vi "DeleteEmptyFolders.vi"() -> ()   [LabVIEW 2020]
uses:
  <resource>/dialog/lvconfig.llb/LV Config Read String.vi
  <userlib>/_MGI/Application Control/MGI Gray if/MGI Gray if False.vi
panel:
  in  "ButtonDelete":bool
  out "FoldersToExclude":string[](array[string])
  out "ContainsEmptyFolder(s)?":bool
  in  "Root Path":path
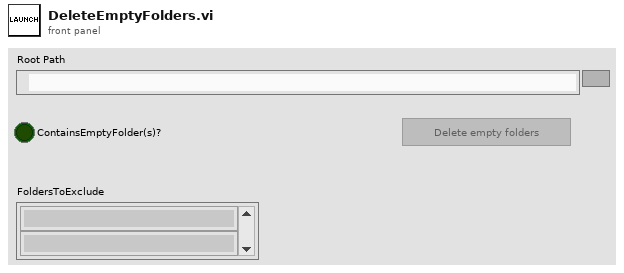
[diagram p1: front panel]
types:
  T1 = enum8{"Enabled", "Disabled", "Disabled and Grayed Out"}
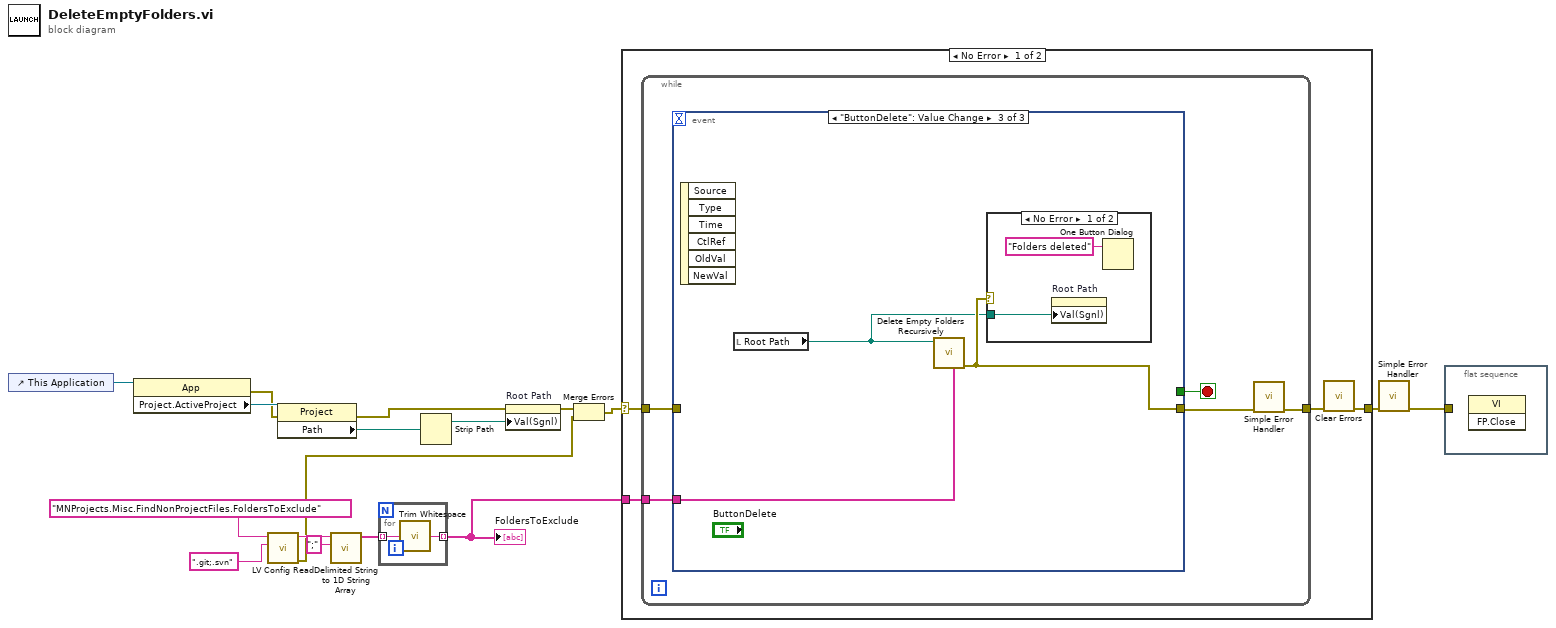
[diagram p0: block diagram]
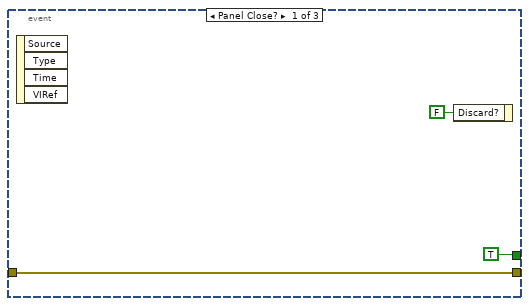
[diagram p2: hidden frame]
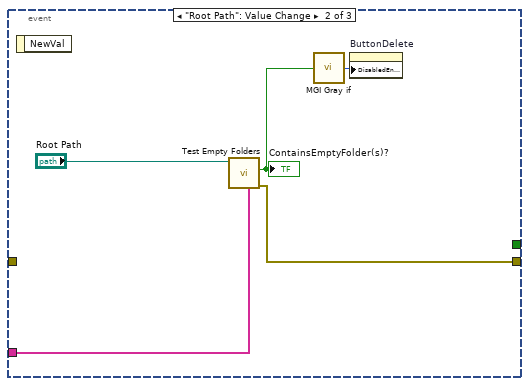
[diagram p3: hidden frame]
diagram:
  n1 = control-ref of="This Application"() -> (w17:refnum<vi>)
  n2 = property class="App"(reference=w17) -> (error out=w13:errorcluster, "Project.ActiveProject"=w16:refnum<vi>)  [unwired: 1 in, 1 out]
  n3 = call-poly <resource>:"LV Config Read.vi"("default value"=".git;.svn", "key"="MNProjects.Misc.FindNonProjectFiles.FoldersToExclude") -> ("error out"=w1:errorcluster, "value"=w7:string)  [unwired: 3 in, 1 out]
  n4 = property class="Project"(reference=w16, error in=w13) -> (error out=w11:errorcluster, "Path"=w15:path)  [unwired: 1 out]
  n5 = call <vilib>:"Delimited String to 1D String Array.vi"("delimiter"=";", "delimited string"=w7) -> ("string array"=w4:string[])  [unwired: 9 in]
  n6 = for {
    tunnel: w4 -> [w19] mode=indexing
    tunnel: [w18] -> w3 mode=indexing
    n7 = call <vilib>:"Trim Whitespace.vi"("string"=w19) -> ("trimmed string"=w18:string)  [unwired: 1 in]
  }
  "FoldersToExclude" <- w3
  n8 = Strip Path(path=w15) -> (stripped path=w10:path)  [unwired: 1 out]
  n9 = property on="Root Path" class="Path"(error in=w11, "Val(Sgnl)"=w10) -> (error out=w9:errorcluster)  [unwired: 1 in, 1 out]
  n10 = Merge Errors(w9, w1) -> (w2:errorcluster)
  n11 = case shown="No Error" w2 {
    selector: w2 -> [w23 w42]
    tunnel: [w20 w42] -> w12
    tunnel: w3 -> [w22 _]
    frame No Error {
      n12 = while {
        tunnel: [w25] -> w21
        tunnel: w23 -> [w27]
        tunnel: w22 -> [w24]
        stop <- w28 stop-if-true
        n13 = event shown="[2] \"ButtonDelete\": Value Change" {
          selector: _ -> [_ _ _]
          dyn-events: _ -> [_ _ _]
          timeout: _ -> [_ _ _]
          tunnel: [TRUE _ _] -> w28
          tunnel: [w29 w35 w38] -> w26
          tunnel: w27 -> [w29 _ _]
          tunnel: w24 -> [_ w34 w39]
          event Panel Close? {
            n14 = event-data() -> ()  [unwired: 1 in, 4 out]
            n15 = event-data("Discard?"=FALSE) -> ()  [unwired: 1 in, 1 out]
          }
          event "Root Path": Value Change {
            n16 = event-data() -> ()  [unwired: 1 in, 1 out]
            n17 = call "Test Empty Folders.vi"("Folders to Exclude"=w34, "Folder Path"="Root Path") -> ("error out"=w35:errorcluster, "ContainsEmptyFolder(s)?"=w32:bool)  [unwired: 8 in]
            "ContainsEmptyFolder(s)?" <- w32
            n18 = call-poly <userlib>:"MGI Gray if.vi"("Boolean"=w32) -> ("Disabled"=w33:T1)
            n19 = property on="ButtonDelete" class="Bool"("DisabledEnum"=w33) -> ()  [unwired: 2 in, 2 out]
          }
          event "ButtonDelete": Value Change {
            n20 = event-data() -> ()  [unwired: 1 in, 6 out]
            n21 = local read "Root Path"() -> (w37:path)
            n22 = call "Delete Empty Folders Recursively.vi"("Folders to Exclude"=w39, "Folder Path"=w37) -> ("error out"=w38:errorcluster)  [unwired: 9 in]
            n23 = case shown="No Error" w38 {
              tunnel: w37 -> [w40 _]
              frame No Error {
                n24 = property on="Root Path" class="Path"("Val(Sgnl)"=w40) -> ()  [unwired: 2 in, 2 out]
                n25 = One Button Dialog(message="Folders deleted") -> ()  [unwired: 1 in, 1 out]
              }
              frame Error {
              }
            }
          }
        }
        n26 = call <vilib>:"Simple Error Handler.vi"("error in (no error)"=w26) -> ("error out"=w25:errorcluster)  [unwired: 4 in, 4 out]
      }
      n27 = call <vilib>:"Clear Errors.vi"("error in (no error)"=w21) -> ("error out"=w20:errorcluster)  [unwired: 5 in, 1 out]
    }
    frame Error {
    }
  }
  n28 = call <vilib>:"Simple Error Handler.vi"("error in (no error)"=w12) -> ("error out"=w14:errorcluster)  [unwired: 4 in, 4 out]
  n29 = flat-sequence {
    tunnel: w14 -> [_]
    frame #0 {
      n30 = invoke class="VI" method="FP.Close"() -> ()  [unwired: 3 in, 3 out]
    }
  }
